vi "DeleteMe.vi"() -> ()   [LabVIEW 2016]
uses:
  DAQLoop_Typedef.ctl
panel:
  out "Array 4":i32[](array[numeric])
  out "Array 3":string[](array[combo])
  in  "stop":bool
  in  "Array 2":string[](array[combo])
  out "Array":string[](array[string])
  out "error out":errorcluster
  in  "error in (no error)":errorcluster
  in  "Cluster":T1
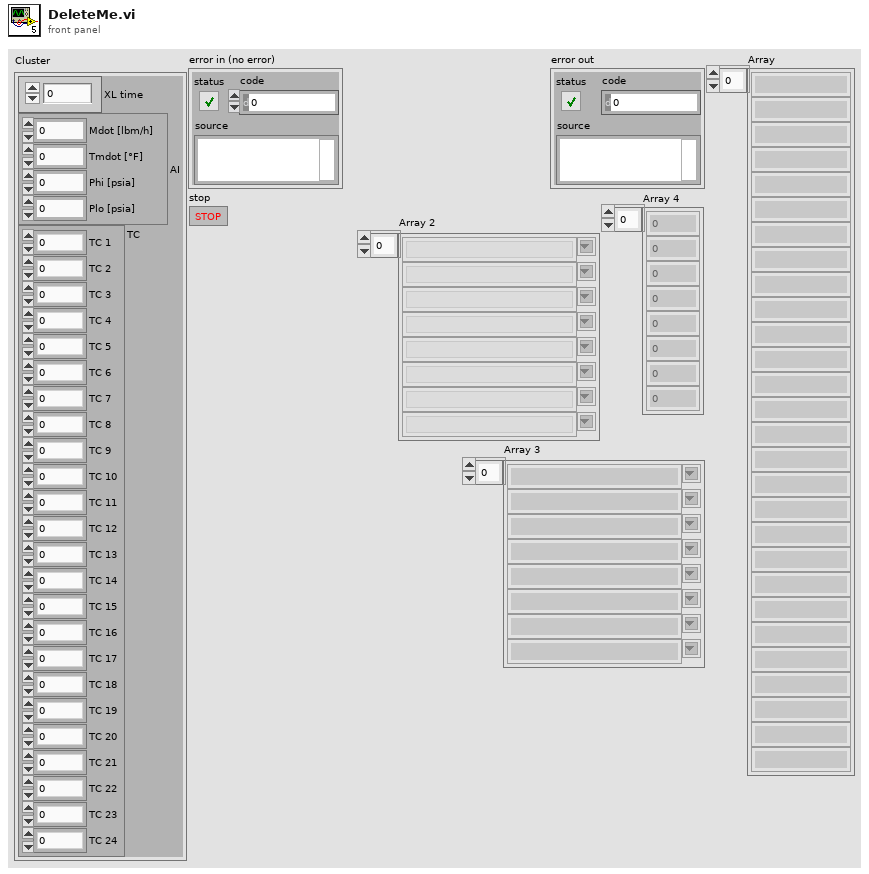
[diagram p1: front panel]
types:
  T1 = typedef "DAQLoop_Typedef.ctl" = cluster{"XL time":dbl, "AI":cluster{"Mdot [lbm/h]":dbl, "Tmdot [°F]":dbl, "Phi [psia]":dbl, "Plo [psia]":dbl}, "TC":cluster{"TC 1":dbl, "TC 2":dbl, "TC 3":dbl, "TC 4":dbl, "TC 5":dbl, "TC 6":dbl, "TC 7":dbl, "TC 8":dbl, "TC 9":dbl, "TC 10":dbl, "TC 11":dbl, "TC 12":dbl, "TC 13":dbl, "TC 14":dbl, "TC 15":dbl, "TC 16":dbl, "TC 17":dbl, "TC 18":dbl, "TC 19":dbl, "TC 20":dbl, "TC 21":dbl, "TC 22":dbl, "TC 23":dbl, "TC 24":dbl}}
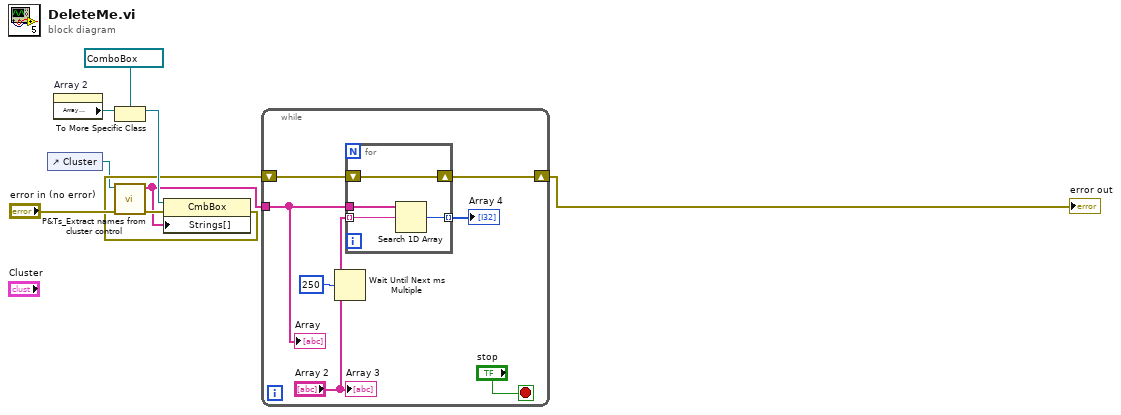
[diagram p0: block diagram]
diagram:
  n1 = control-ref of="Cluster"() -> (w4:refnum<vi>)
  n2 = property on="Array 2" class="Arr (strict)"() -> ("Array Element"=w8:refnum<vi>)  [unwired: 2 in, 2 out]
  n3 = To More Specific Class(target class=refnum<vi> refnum ("Combo Box"), reference=w8) -> (specific class reference=w7:refnum<vi>)  [unwired: 1 in, 1 out]
  n4 = call "P&Ts_Extract names from cluster control.vi"("error in (no error)"="error in (no error)", "Cluster 2"=w4) -> ("error out"=w3:errorcluster, "Array"=w2:string[])  [unwired: 8 in]
  n5 = property class="CmbBox"(reference=w7, error in=w3, "Strings[]"=w2) -> (error out=w5:errorcluster)  [unwired: 1 out]
  n6 = while {
    shift-right: [w14] -> w1
    shift-left: w5 -> [w12]
    tunnel: w2 -> [w11]
    stop <- "stop" stop-if-true
    n7 = Wait Until Next ms Multiple(millisecond multiple=u32 250) -> ()  [unwired: 1 out]
    n8 = for {
      shift-right: [w20] -> w14
      shift-left: w12 -> [w20]
      tunnel: "Array 2" -> [w18] mode=indexing
      tunnel: w11 -> [w19]
      tunnel: [w17] -> w10 mode=indexing
      n9 = Search 1D Array(1D array=w19, element=w18) -> (index of element=w17:i32)  [unwired: 1 in]
    }
    "Array 4" <- w10
    "Array 3" <- "Array 2"
    "Array" <- w11
  }
  "error out" <- w1
